vi "Set_Field_AMI.vi"() -> ()   [LabVIEW 2016]
uses:
  Global/Global Variables/Data_Display_global.vi
  Global/Global Variables/global.vi
panel:
  in  "Cancel Button":bool
  in  "OK Button":bool
  in  "Rate":dbl
  in  "AMI Setpoint Phi(Deg)":dbl
  in  "AMI Setpoint B(T)":dbl
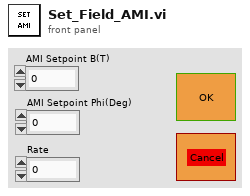
[diagram p1: front panel]
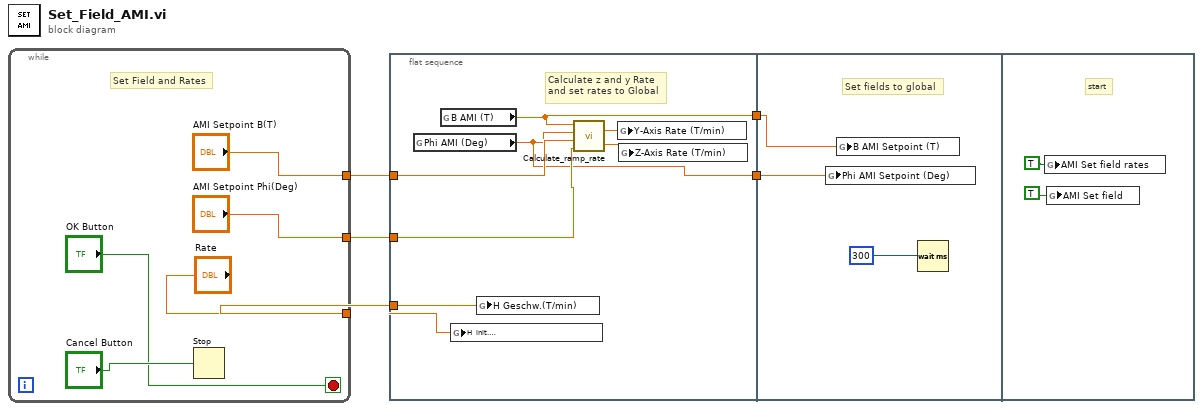
[diagram p0: block diagram]
diagram:
  n1 = while {
    tunnel: ["AMI Setpoint B(T)"] -> w5
    tunnel: ["AMI Setpoint Phi(Deg)"] -> w4
    tunnel: ["Rate"] -> w3
    stop <- "OK Button" stop-if-true
    # "Set Field and Rates"
    n2 = Stop(stop? (T)="Cancel Button") -> ()
  }
  n3 = flat-sequence {
    tunnel: w5 -> [w15]
    tunnel: w4 -> [w14]
    tunnel: w3 -> [w13]
    tunnel: [w12] -> w2
    tunnel: [w11] -> w1
    tunnel: w2 -> [w20]
    tunnel: w1 -> [w19]
    frame #0 {
      # "Calculate z and y Rate\nand set rates to Global"
      n4 = global read "Data_Display_global.vi" "Phi AMI (Deg)"() -> (w11:dbl)
      n5 = global read "Data_Display_global.vi" "B AMI (T)"() -> (w12:dbl)
      n6 = global write "global.vi" "H  init. \nGeschw.(T/min)"(w13) -> ()
      n7 = global write "global.vi" "H Geschw.(T/min)"(w13) -> ()
      n8 = call "Calculate_ramp_rate.vi"("Phi (Deg)"=w14, "H_final (T)"=w15, "Phi_init (Deg)"=w11, "H_init (T)"=w12) -> ("Z-Ramp"=w16:dbl, "Y-Ramp"=w17:dbl)  [unwired: 2 in]
      n9 = global write "Data_Display_global.vi" "Y-Axis Rate (T/min)"(w17) -> ()
      n10 = global write "Data_Display_global.vi" "Z-Axis Rate (T/min)"(w16) -> ()
    }
    frame #1 {
      # "Set fields to global"
      n11 = global write "Data_Display_global.vi" "Phi AMI Setpoint (Deg)"(w19) -> ()
      n12 = global write "Data_Display_global.vi" "B AMI Setpoint (T)"(w20) -> ()
      n13 = Wait (ms)(milliseconds to wait=300) -> ()  [unwired: 1 out]
    }
    frame #2 {
      # "start"
      n14 = global write "Data_Display_global.vi" "AMI Set field rates"(TRUE) -> ()
      n15 = global write "Data_Display_global.vi" "AMI Set field"(TRUE) -> ()
    }
  }
